vi "VCS Get Inc Encoder Parameter.vi"(0 "axis in":cluster{"keyHandle":u32, "nodeId":u16}={"keyHandle"=0, "nodeId"=1}, 11 "error in (no error)":errorcluster) -> (4 "axis out":cluster{"keyHandle":u32, "nodeId":u16}={"keyHandle"=0, "nodeId"=1}, 8 "incremental encoder parameter":T1, 15 "error out":errorcluster)   [LabVIEW 2019, in "maxonEPOS.lvlib"]
doc: "With function <B>VCS_GetIncEncoderParameter</B> it is possible to read the incremental encoder parameters."
uses:
  Examples/maxonEPOS.lvlib
  Resources/EposCmd.dll
  Resources/EposCmd64.dll
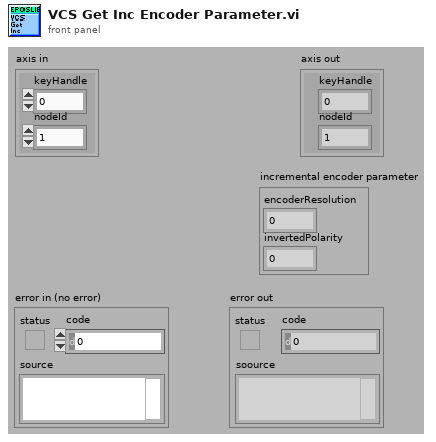
[diagram p1: front panel]
types:
  T1 = cluster{"encoderResolution":u32, "invertedPolarity":i32}
  T2 = cluster{"pEncoderResolution":u32, "pInvertedPolarity":i32}
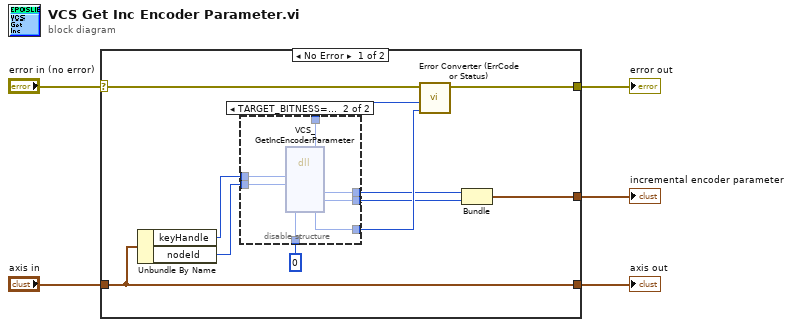
[diagram p0: block diagram]
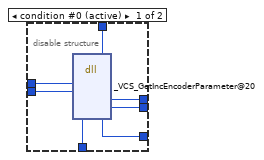
[diagram p2: hidden frame]
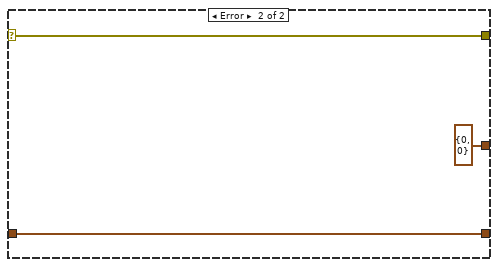
[diagram p3: hidden frame]
diagram:
  n1 = case shown="No Error" "error in (no error)" {
    selector: "error in (no error)" -> [w14 w32]
    tunnel: "axis in" -> [w16 w33]
    tunnel: [w16 w33] -> w4
    tunnel: [w15 w32] -> w3
    tunnel: [w6 T2 {"pEncoderResolution"=0, "pInvertedPolarity"=0}] -> w1
    frame No Error {
      n2 = Unbundle By Name(w16) -> ("keyHandle"=w10:u32, "nodeId"=w9:u16)
      n3 = disable-structure shown="TARGET_BITNESS==64" {
        disable-tunnel: u32 0 ("pErrorCode") -> [w23 w30]
        disable-tunnel: [w22 w29] -> w12
        disable-tunnel: [w21 w28] -> w11
        disable-tunnel: w10 -> [w20 w27]
        disable-tunnel: w9 -> [w19 w26]
        disable-tunnel: [w18 w25] -> w8
        disable-tunnel: [w17 w24] -> w7
        frame condition #0 (active) {
          n4 = dll-call lib="C:/workspace/project/scancon/sw/SSI_Tool/InstrumentsInterfaces/Motordriver/maxon EPOS/Resources/EposCmd.*" fn="_VCS_GetIncEncoderParameter@20"("KeyHandle"=w20, "NodeId"=w19, "pErrorCode"=w23) -> (w22:i32, "pEncoderResolution"=w18:u32, "pInvertedPolarity"=w17:i32, "pErrorCode"=w21:u32)  [unwired: 7 in, 2 out]
        }
        frame condition #1 {
          n5 = dll-call lib="C:/Sources/LabView/maxon EPOS/Resources/EposCmd64.*" fn="VCS_GetIncEncoderParameter" ("EposCmd.dll:_VCS_GetIncEncoderParameter@20")("KeyHandle"=w27, "NodeId"=w26, "pErrorCode"=w30) -> ("Rückgabetyp"=w29:i32, "pEncoderResolution"=w25:u32, "pInvertedPolarity"=w24:i32, "pErrorCode"=w28:u32)  [unwired: 7 in, 2 out]
        }
      }
      n6 = call "Error Converter (ErrCode or Status).vi"("error code"=w11, "return type"=w12, "error in (no error)"=w14) -> ("error out"=w15:errorcluster)  [unwired: 7 in]
      n7 = Bundle("pEncoderResolution"=w8, "pInvertedPolarity"=w7) -> (w6:T2)  [unwired: 1 in]
    }
    frame Error {
    }
  }
  "error out" <- w3
  "axis out" <- w4
  "incremental encoder parameter" <- w1
